vi "Convert Array to AcquireParams.vi"(1 "ACQUIPARAMS BYTE ARRAY":u32[](array[numeric])) -> (0 "ACQUIPARAMS":T1 {"CFA"."CFA" items=["CFA_NONE", "CFA_VRI", "CFA_VRIV6", "CFA_BAYER", "CFA_BAYERFLIP"]; "TriggerTime"."fractions" format="%32.0f"})   [LabVIEW 2013, in "VRI.lvlib"]
doc: "This VI is used to convert an array of U32 to theAcquirParams cluster. This is needed because the DLL function cannot return the cluster directly."
uses:
  VRI.lvlib
  _Type Defs/PHCon ACQUIPARAMS.ctl
  _Type Defs/PhCon SyncImaging.ctl
  _Type Defs/Rect.ctl
  _Type Defs/PHCon Time64.ctl
  _Type Defs/PhInt CFA.ctl
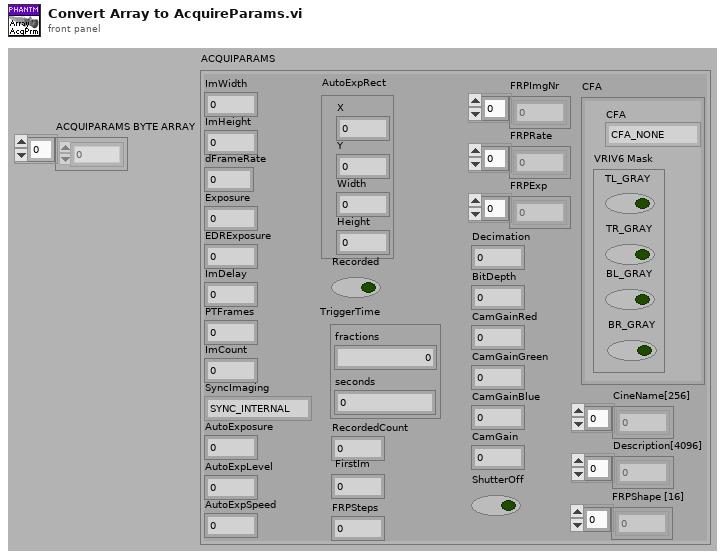
[diagram p1: front panel]
types:
  T1 = typedef "VRI.lvlib/PHCon ACQUIPARAMS.ctl" = cluster{"ImWidth":u32, "ImHeight":u32, "(deprecated)FrameRateInt":u32, "Exposure":u32, "EDRExposure":u32, "ImDelay":u32, "PTFrames":u32, "ImCount":u32, "SyncImaging":T2, "AutoExposure":u32, "AutoExpLevel":u32, "AutoExpSpeed":u32, "AutoExpRect":T3, "Recorded":bool, "TriggerTime":T4, "RecordedCount":u32, "FirstIm":i32, "FRPSteps":u32, "FRPImgNr":i32[], "FRPRate":u32[], "FRPExp":u32[], "Decimation":u32, "BitDepth":u32, "CamGainRed":u32, "CamGainGreen":u32, "CamGainBlue":u32, "CamGain":u32, "ShutterOff":bool, "CFA":T5, "CineName[256]":u8[], "Description[4096]":u8[], "FRPShape [16]":u32[], "dFrameRate":dbl}
  T2 = typedef "VRI.lvlib/PhCon SyncImaging.ctl" = enum32{"SYNC_INTERNAL", "SYNC_EXTERNAL", "SYNC_LOCKTOIRIG"}
  T3 = typedef "VRI.lvlib/Rect.ctl" = cluster{"X":i32, "Y":i32, "Width":i32, "Height":i32}
  T4 = typedef "VRI.lvlib/PHCon Time64.ctl" = cluster{"fractions":u32, "seconds":u32}
  T5 = typedef "VRI.lvlib/PhInt CFA.ctl" = cluster{"CFA":u32, "VRIV6 Mask":cluster{"TL_GRAY":bool, "TR_GRAY":bool, "BL_GRAY":bool, "BR_GRAY":bool}}
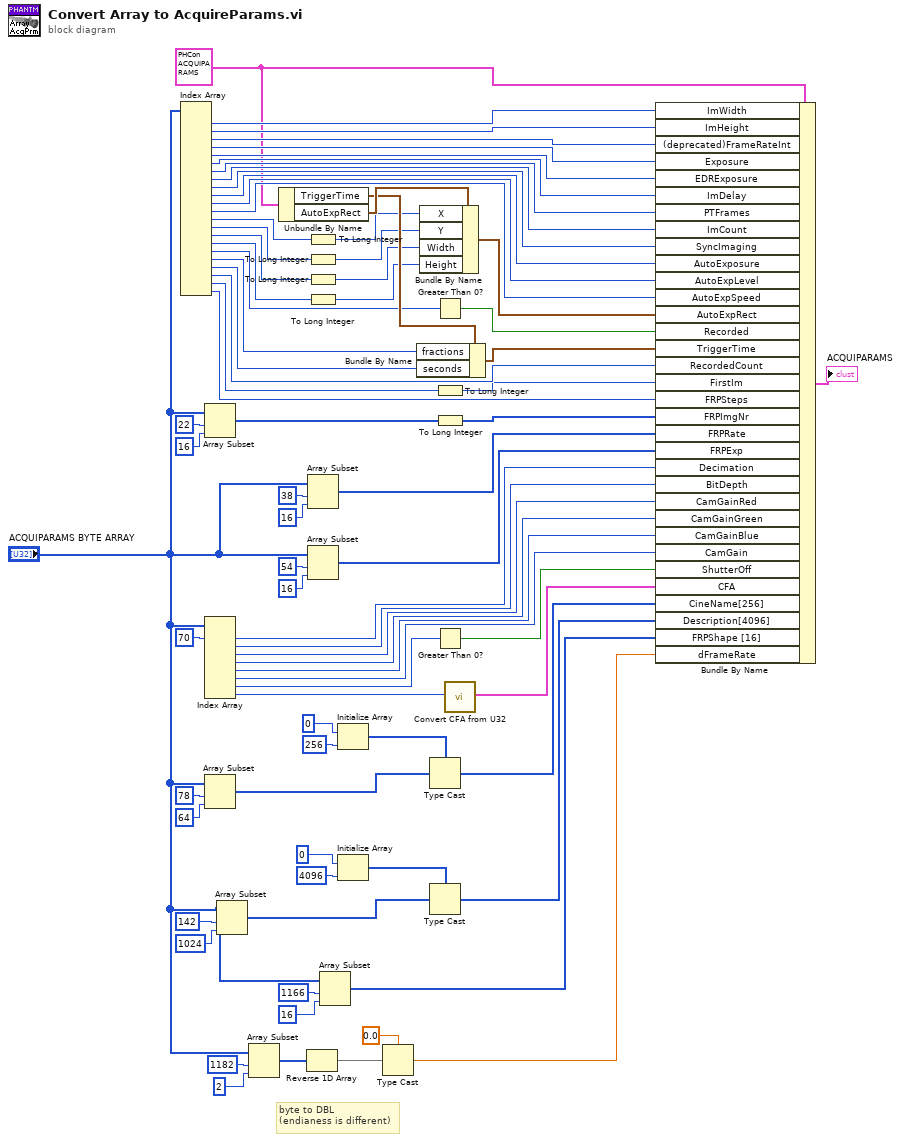
[diagram p0: block diagram]
diagram:
  w67 = T1 {"ImWidth"=0, "ImHeight"=0, "(deprecated)FrameRateInt"=0, "Exposure"=0, "EDRExposure"=0, "ImDelay"=0, "PTFrames"=0, "ImCount"=0, "SyncImaging"=enum."SYNC_INTERNAL", "AutoExposure"=0, "AutoExpLevel"=0, "AutoExpSpeed"=0, "AutoExpRect"={"X"=0, "Y"=0, "Width"=0, "Height"=0}, "Recorded"=FALSE, "TriggerTime"={"fractions"=0, "seconds"=0}, "RecordedCount"=0, "FirstIm"=0, "FRPSteps"=0, "FRPImgNr"=[], "FRPRate"=[], "FRPExp"=[], "Decimation"=0, "BitDepth"=0, "CamGainRed"=0, "CamGainGreen"=0, "CamGainBlue"=0, "CamGain"=0, "ShutterOff"=FALSE, "CFA"={"CFA"=0, "VRIV6 Mask"={"TL_GRAY"=FALSE, "TR_GRAY"=FALSE, "BL_GRAY"=FALSE, "BR_GRAY"=FALSE}}, "CineName[256]"=[], "Description[4096]"=[], "FRPShape [16]"=[], "dFrameRate"=0.0} ("ACQUIPARAMS")
  # "byte to DBL\n(endianess is different)"
  n1 = Index Array(array="ACQUIPARAMS BYTE ARRAY") -> (element #1=w79:u32, element #2=w78:u32, element #3=w77:u32, element #4=w76:u32, element #5=w75:u32, element #6=w74:u32, element #7=w73:u32, element #8=w72:u32, element #9=w71:u32, element #10=w70:u32, element #11=w69:u32, element #12=w68:u32, element #13=w64:u32, element #14=w63:u32, element #15=w62:u32, element #16=w61:u32, element #17=w51:u32, element #18=w50:u32, element #19=w49:u32, element #20=w48:u32, element #21=w47:u32, element #22=w45:u32)  [unwired: 22 in]
  n2 = Array Subset(array="ACQUIPARAMS BYTE ARRAY", index=22, length=16) -> (w40:u32[])
  n3 = Index Array(array="ACQUIPARAMS BYTE ARRAY", index #1=70 ("index")) -> (element #1=w31:u32, element #2=w30:u32, element #3=w29:u32, element #4=w28:u32, element #5=w27:u32, element #6=w26:u32, element #7=w25:u32, element #8=w12:u32)  [unwired: 7 in]
  n4 = Array Subset(array="ACQUIPARAMS BYTE ARRAY", index=78, length=64) -> (w21:u32[])
  n5 = Array Subset(array="ACQUIPARAMS BYTE ARRAY", index=142, length=1024) -> (w14:u32[])
  n6 = Array Subset(array="ACQUIPARAMS BYTE ARRAY", index=1182, length=2) -> (w4:u32[])
  n7 = Unbundle By Name(w67) -> ("TriggerTime"=w60:T4, "AutoExpRect"=w66:T3)
  n8 = Reverse 1D Array(array=w4) -> (reversed array=w1:u32[])
  n9 = To Long Integer(number=w64) -> (32bit integer=w59:i32)
  n10 = To Long Integer(number=w63) -> (32bit integer=w58:i32)
  n11 = To Long Integer(number=w62) -> (32bit integer=w57:i32)
  n12 = To Long Integer(number=w61) -> (32bit integer=w56:i32)
  n13 = Array Subset(array="ACQUIPARAMS BYTE ARRAY", index=38, length=16) -> (w36:u32[])
  n14 = Array Subset(array="ACQUIPARAMS BYTE ARRAY", index=54, length=16) -> (w33:u32[])
  n15 = Array Subset(array="ACQUIPARAMS BYTE ARRAY", index=1166, length=16) -> (w8:u32[])
  n16 = Initialize Array(u8 0 ("element"), 256 ("dimension size")) -> (w41:u8[])
  n17 = Initialize Array(u8 0 ("element"), 4096 ("dimension size")) -> (w15:u8[])
  n18 = Type Cast(type=0.0 ("length"), x=w1) -> (*(type *) &x=w3:dbl)
  n19 = Bundle By Name(cluster=w60, "fractions"=w50, "seconds"=w49) -> (w53:T4)
  n20 = Bundle By Name(cluster=w66, "X"=w59, "Y"=w58, "Width"=w57, "Height"=w56) -> (w65:T3)
  n21 = Type Cast(type=w41, x=w21) -> (*(type *) &x=w20:u8[])
  n22 = Type Cast(type=w15, x=w14) -> (*(type *) &x=w13:u8[])
  n23 = Greater Than 0?(x=w51) -> (x > 0?=w52:bool)
  n24 = To Long Integer(number=w47) -> (32bit integer=w46:i32)
  n25 = To Long Integer(number=w40) -> (32bit integer=w39:i32[])
  n26 = Greater Than 0?(x=w25) -> (x > 0?=w24:bool)
  n27 = call "Convert CFA from U32.vi"("CFA in"=w12) -> ("CFA"=w11:T5)  [unwired: 18 out]
  n28 = Bundle By Name(cluster=w67, "ImWidth"=w79, "ImHeight"=w78, "(deprecated)FrameRateInt"=w77, "Exposure"=w76, "EDRExposure"=w75, "ImDelay"=w74, "PTFrames"=w73, "ImCount"=w72, "SyncImaging"=w71, "AutoExposure"=w70, "AutoExpLevel"=w69, "AutoExpSpeed"=w68, "AutoExpRect"=w65, "Recorded"=w52, "TriggerTime"=w53, "RecordedCount"=w48, "FirstIm"=w46, "FRPSteps"=w45, "FRPImgNr"=w39, "FRPRate"=w36, "FRPExp"=w33, "Decimation"=w31, "BitDepth"=w30, "CamGainRed"=w29, "CamGainGreen"=w28, "CamGainBlue"=w27, "CamGain"=w26, "ShutterOff"=w24, "CFA"=w11, "CineName[256]"=w20, "Description[4096]"=w13, "FRPShape [16]"=w8, "dFrameRate"=w3) -> (→"ACQUIPARAMS":T1)
